vi "oax_Calculate Number of Samples for DIO.vi"(8 "Tacho Pulse/Rev":i32=1 min=0, 9 "sample rate [samples/s]":dbl=10000.0, 10 "number of samples to acquire":i32=10000, 11 "DSA device type":T1 items=["4472"=0, "4474"=10, "4461"=1, "4462"=11, "4464"=12, "449x"=6, "9232"=7, "9233"=2, "9234"=3, "9229"=4, "9239"=5]) -> (3 "number of samples per channel":i32)   [LabVIEW 2017]
doc: "Calculates the number of samples per channel input of the DIO read VI.\nFor 446x/447x and other devices based on PXI platform, the number should be -1, which means reading all the available samples. For cDAQ platform, 9401 requires a specify number of samples to read, otherwise there will be an empty output. For the compensate slow roll examples, the rotating speed must be slow. This VI assumes 600 RPM as the fastest speed."
uses:
  <vilib>/addons/Sound and Vibration/Order Analysis/Example Support/sub VIs/OAXML_DSA Device Type.ctl
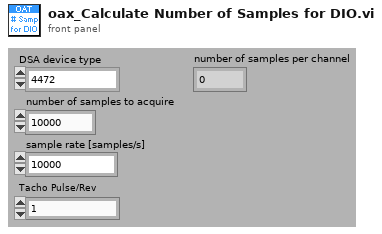
[diagram p1: front panel]
types:
  T1 = typedef "OAXML_DSA Device Type.ctl" = u16
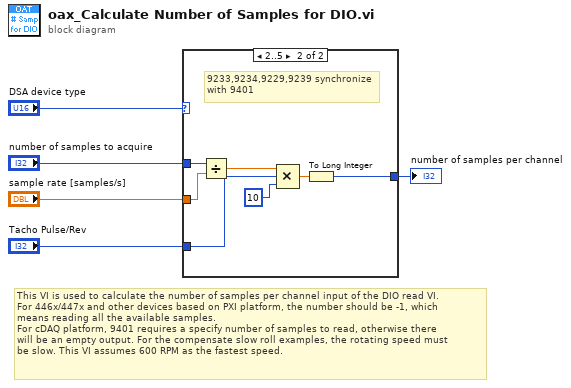
[diagram p0: block diagram]
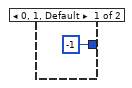
[diagram p2: hidden frame]
diagram:
  # "This VI is used to calculate the number of samples per channel input of the DIO read VI.\nFor 446x/447x and other devices based on PXI platform, the number should be -1, which\nmeans reading all the available samples.\nFor cDAQ platform, 9401 requires a specify number of samples to read, otherwise there\nwill be an empty output. For the compensate slow roll examples, the rotating speed must\nbe slow. This VI assumes 600 RPM as the fastest speed."
  n1 = case shown="2..5" "DSA device type" {
    tunnel: "number of samples to acquire" -> [_ w13]
    tunnel: "sample rate [samples/s]" -> [_ w12]
    tunnel: "Tacho Pulse/Rev" -> [_ w10]
    tunnel: [-1 w7] -> w1
    frame 0, 1, Default {
    }
    frame 2..5 {
      # "9233,9234,9229,9239 synchronize\nwith 9401"
      n2 = Divide(x=w13, y=w12) -> (x/y=w11:dbl)
      n3 = Compound Arithmetic op=MULTIPLY(w11, w10, 10 ("Tacho Pulse/Rev")) -> (w8:dbl)
      n4 = To Long Integer(number=w8) -> (32bit integer=w7:i32)
    }
  }
  "number of samples per channel" <- w1
